vi "Select Pins by Device Type.vi"(8 "error in (no error)":errorcluster, 9 "Publishable IDs":string[](array[string])=["State00", "State01", "State02", "State04", "State08"], 10 "SP4T_Pins":string[](array[string])=["RF1", "RF2", "RF3", "RF4"], 11 "USID":T1 max=15) -> (0 "error out":errorcluster, 2 "Published ID":string[](array[string]), 3 "Pins to Test":string[][](array[string]))   [LabVIEW 2013]
uses:
  Controls/USID.ctl
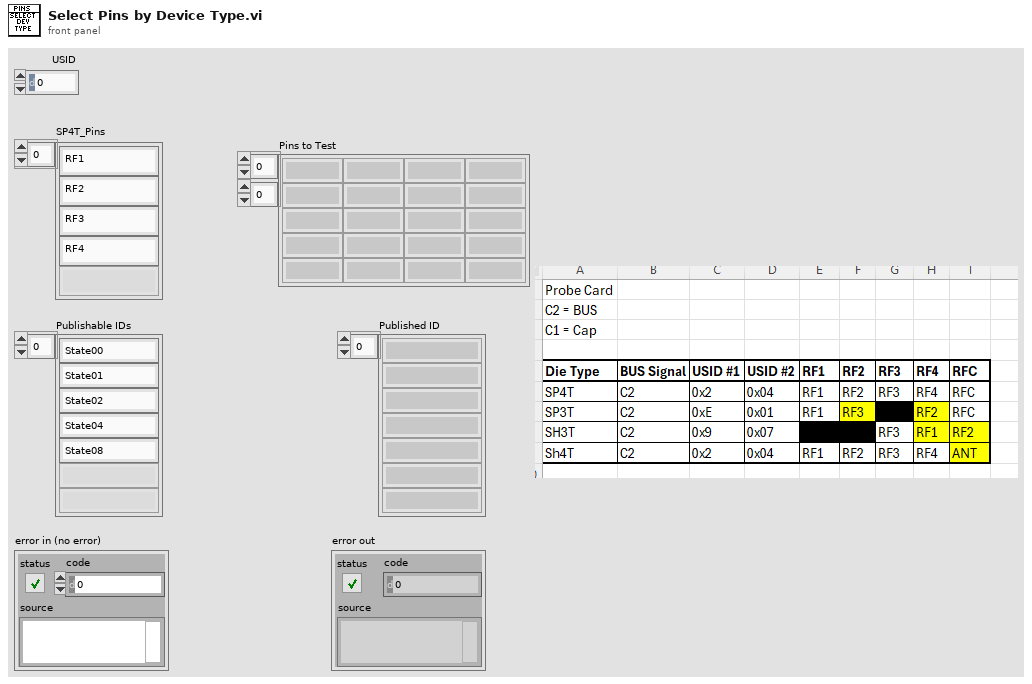
[diagram p1: front panel]
types:
  T1 = typedef "USID.ctl" = u8
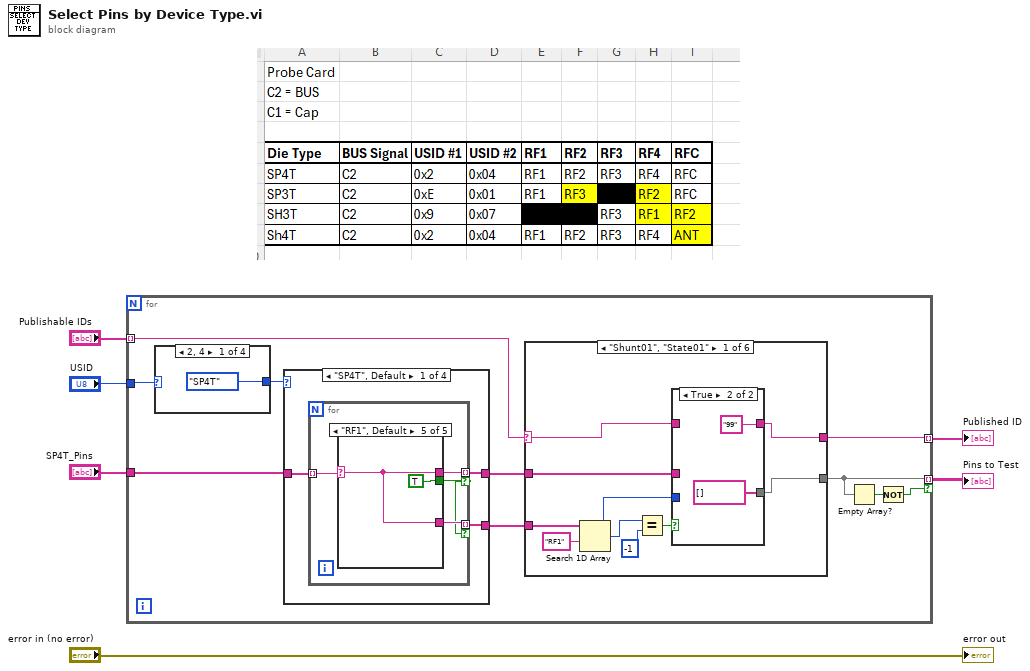
[diagram p0: block diagram]
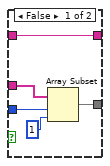
[diagram p2: hidden frame]
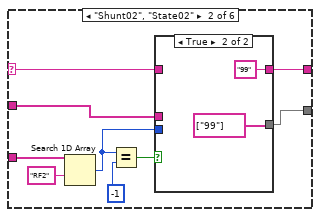
[diagram p3: hidden frame]
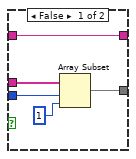
[diagram p4: hidden frame]
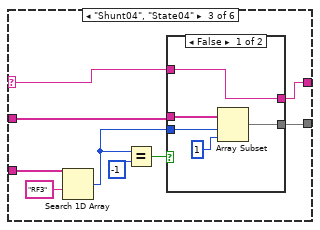
[diagram p5: hidden frame]
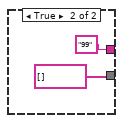
[diagram p6: hidden frame]
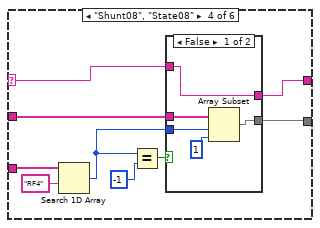
[diagram p7: hidden frame]
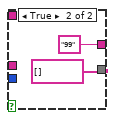
[diagram p8: hidden frame]
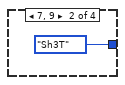
[diagram p11: hidden frame]
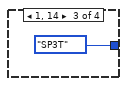
[diagram p12: hidden frame]
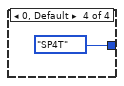
[diagram p13: hidden frame]
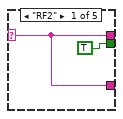
[diagram p14: hidden frame]
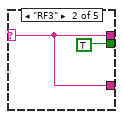
[diagram p15: hidden frame]
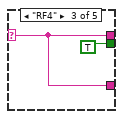
[diagram p16: hidden frame]
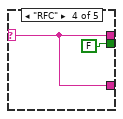
[diagram p17: hidden frame]
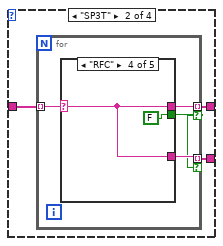
[diagram p18: hidden frame]
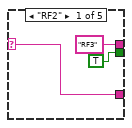
[diagram p19: hidden frame]
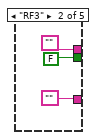
[diagram p20: hidden frame]
diagram:
  n1 = for {
    tunnel: "Publishable IDs" -> [w13] mode=indexing
    tunnel: "USID" -> [w15]
    tunnel: "SP4T_Pins" -> [w14]
    tunnel: [w9] -> w2 mode=indexing if=w7
    tunnel: [w10] -> w3 mode=indexing
    n2 = case shown="2, 4" w15 {
      tunnel: [enum16{"SP4T", "SP3T", "Sh3T", "Sh4T"}."SP4T" ("Die Type 2") enum16{"SP4T", "SP3T", "Sh3T", "Sh4T"}."Sh3T" ("Die Type 2") enum16{"SP4T", "SP3T", "Sh3T", "Sh4T"}."SP3T" ("Die Type 2") enum16{"SP4T", "SP3T", "Sh3T", "Sh4T"}."SP4T" ("Die Type 2")] -> w16
      frame 2, 4 {
      }
      frame 7, 9 {
      }
      frame 1, 14 {
      }
      frame 0, Default {
      }
    }
    n3 = case shown="\"SP4T\", Default" w16 {
      tunnel: w14 -> [w91 w108 w128 w147]
      tunnel: [w90 w107 w127 w146] -> w11
      tunnel: [w89 w106 w126 w145] -> w12
      frame "SP4T", Default {
        n4 = for {
          tunnel: [w95] -> w90 mode=indexing if=w93
          tunnel: [w94] -> w89 mode=indexing if=w93
          tunnel: w91 -> [w92] mode=indexing
          n5 = case shown="\"RF1\", Default" w92 {
            selector: w92 -> [w96 w98 w100 w102 w104]
            tunnel: [w96 w98 w100 w102 w104] -> w95
            tunnel: [TRUE TRUE TRUE FALSE TRUE] -> w93
            tunnel: [w96 w98 w100 w102 w104] -> w94
            frame "RF2" {
            }
            frame "RF3" {
            }
            frame "RF4" {
            }
            frame "RFC" {
            }
            frame "RF1", Default {
            }
          }
        }
      }
      frame "SP3T" {
        n6 = for {
          tunnel: w108 -> [w112] mode=indexing
          tunnel: [w111] -> w107 mode=indexing if=w109
          tunnel: [w110] -> w106 mode=indexing if=w109
          n7 = case shown="\"RFC\"" w112 {
            selector: w112 -> [w113 _ w119 w122 w124]
            tunnel: ["RF3" "" "RF2" w122 w124] -> w111
            tunnel: [TRUE FALSE TRUE FALSE TRUE] -> w109
            tunnel: [w113 "" w119 w122 w124] -> w110
            frame "RF2" {
            }
            frame "RF3" {
            }
            frame "RF4" {
            }
            frame "RFC" {
            }
            frame "RF1", Default {
            }
          }
        }
      }
      frame "Sh3T" {
        n8 = for {
          tunnel: w128 -> [w132] mode=indexing
          tunnel: [w131] -> w127 mode=indexing if=w129
          tunnel: [w130] -> w126 mode=indexing if=w129
          n9 = case shown="\"RFC\"" w132 {
            selector: w132 -> [w133 w135 w137 w142 w143]
            tunnel: [w133 w135 w137 w142 w143] -> w131
            tunnel: [FALSE TRUE TRUE TRUE FALSE] -> w129
            tunnel: [w133 w135 "RF1" "RF2" w143] -> w130
            frame "RF2" {
            }
            frame "RF3" {
            }
            frame "RF4" {
            }
            frame "RFC" {
            }
            frame "RF1", Default {
            }
          }
        }
      }
      frame "Sh4T" {
        n10 = for {
          tunnel: w147 -> [w151] mode=indexing
          tunnel: [w150] -> w146 mode=indexing if=w148
          tunnel: [w149] -> w145 mode=indexing if=w148
          n11 = case shown="\"RFC\"" w151 {
            selector: w151 -> [w152 w154 w156 w160 w161]
            tunnel: [w152 w154 w156 w160 w161] -> w150
            tunnel: [TRUE TRUE TRUE TRUE TRUE] -> w148
            tunnel: [w152 w154 w156 "ANT" w161] -> w149
            frame "RF2" {
            }
            frame "RF3" {
            }
            frame "RF4" {
            }
            frame "RFC" {
            }
            frame "RF1", Default {
            }
          }
        }
      }
    }
    n12 = case shown="\"Shunt01\", \"State01\"" w13 {
      selector: w13 -> [w20 w36 w50 w67 w81 w83]
      tunnel: [w18 w33 w54 w69 w82 w84] -> w9
      tunnel: w12 -> [w21 w34 w55 w65 _ _]
      tunnel: w11 -> [w17 w35 w56 w66 w82 w84]
      tunnel: [w19 w37 w49 w68 w81 w83] -> w10
      frame "Shunt01", "State01" {
        n13 = Search 1D Array(1D array=w21, element="RF1") -> (index of element=w24:i32)  [unwired: 1 in]
        n14 = Equal?(x=w24, y=-1) -> (x = y?=w22:bool)
        n15 = case shown="True" w22 {
          tunnel: w24 -> [w30 _]
          tunnel: [w27 string[] []] -> w18
          tunnel: [w28 "99"] -> w19
          tunnel: w20 -> [w28 _]
          tunnel: w17 -> [w26 _]
          frame False {
            n16 = Array Subset(array=w26, index=w30, length=1) -> (w27:string[])
          }
          frame True {
          }
        }
      }
      frame "Shunt02", "State02" {
        n17 = Search 1D Array(1D array=w34, element="RF2") -> (index of element=w40:i32)  [unwired: 1 in]
        n18 = Equal?(x=w40, y=-1) -> (x = y?=w38:bool)
        n19 = case shown="True" w38 {
          tunnel: w40 -> [w46 _]
          tunnel: w35 -> [w44 _]
          tunnel: [w43 string[] ["99"]] -> w33
          tunnel: w36 -> [w42 _]
          tunnel: [w42 "99"] -> w37
          frame False {
            n20 = Array Subset(array=w44, index=w46, length=1) -> (w43:string[])
          }
          frame True {
          }
        }
      }
      frame "Shunt04", "State04" {
        n21 = Search 1D Array(1D array=w55, element="RF3") -> (index of element=w53:i32)  [unwired: 1 in]
        n22 = Equal?(x=w53, y=-1) -> (x = y?=w51:bool)
        n23 = case shown="False" w51 {
          tunnel: w53 -> [w62 _]
          tunnel: w56 -> [w60 _]
          tunnel: [w59 string[] []] -> w54
          tunnel: w50 -> [w58 _]
          tunnel: [w58 "99"] -> w49
          frame False {
            n24 = Array Subset(array=w60, index=w62, length=1) -> (w59:string[])
          }
          frame True {
          }
        }
      }
      frame "Shunt08", "State08" {
        n25 = Search 1D Array(1D array=w65, element="RF4") -> (index of element=w72:i32)  [unwired: 1 in]
        n26 = Equal?(x=w72, y=-1) -> (x = y?=w70:bool)
        n27 = case shown="False" w70 {
          tunnel: w72 -> [w78 _]
          tunnel: [w75 string[] []] -> w69
          tunnel: [w76 "99"] -> w68
          tunnel: w67 -> [w76 _]
          tunnel: w66 -> [w74 _]
          frame False {
            n28 = Array Subset(array=w74, index=w78, length=1) -> (w75:string[])
          }
          frame True {
          }
        }
      }
      frame "Shunt15", "State15" {
      }
      frame "Shunt00", "State00", Default {
      }
    }
    n29 = Empty Array?(array=w9) -> (empty?=w8:bool)
    n30 = Not(x=w8) -> (.not. x?=w7:bool)
  }
  "Published ID" <- w3
  "Pins to Test" <- w2
  "error out" <- "error in (no error)"
